vi "SetModelAndSuffix.vi"(5 "Revision":string, 6 "Serial Number":string, 7 "PartNumberData":T1(array[cluster]), 8 "error in (no error)":errorcluster, 9 "Part Number":string, 10 "ArrayIndex":i32=1, 11 "Sequence Context In":refnum<k7>) -> (0 "error out":errorcluster, 3 "Sequence Context Out":refnum<k7>)   [LabVIEW 2021]
uses:
  <vilib>/addons/TestStand/_TSUtility.llb/TestStand - Set Property Value (String).vi
  <vilib>/addons/TestStand/_TSUtility.llb/TestStand - Set Property Value (Boolean).vi
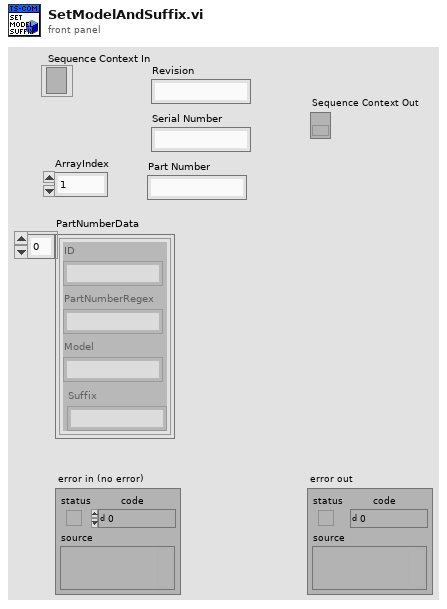
[diagram p1: front panel]
types:
  T1 = cluster{"ID":string, "PartNumberRegex":string, "Model":string, "Suffix":string}[]
  T2 = cluster{"ID":string, "PartNumberRegex":string, "Model":string, "Suffix":string}
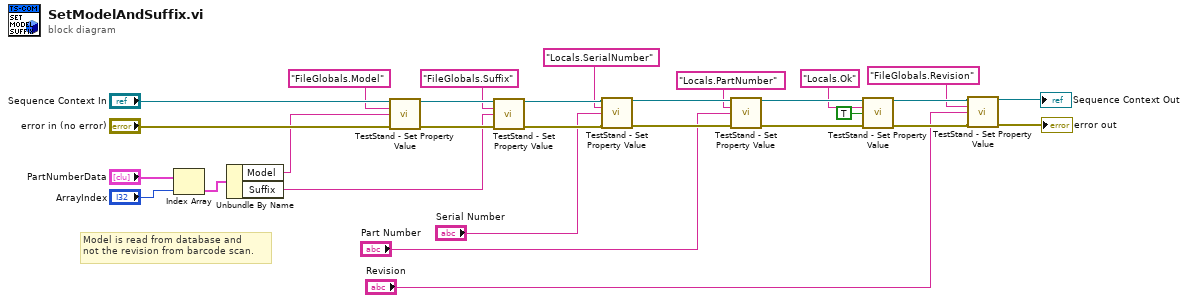
[diagram p0: block diagram]
diagram:
  # "Model is read from database and \nnot the revision from barcode scan."
  n1 = Index Array(array="PartNumberData", index="ArrayIndex") -> (element=w9:T2)
  n2 = Unbundle By Name(w9) -> ("Model"=w7:string, "Suffix"=w8:string)
  n3 = call-poly <vilib>:"TestStand - Set Property Value.vi"("Sequence Context In"="Sequence Context In", "Lookup String"="FileGlobals.Model", "New Value"=w7, "error in (no error)"="error in (no error)") -> ("Sequence Context Out"=w27:refnum<k7>, "error out"=w25:errorcluster)  [unwired: 10 in]
  n4 = call-poly <vilib>:"TestStand - Set Property Value.vi"("Sequence Context In"=w27, "Lookup String"="FileGlobals.Suffix", "New Value"=w8, "error in (no error)"=w25) -> ("Sequence Context Out"=w23:refnum<k7>, "error out"=w22:errorcluster)  [unwired: 10 in]
  n5 = call-poly <vilib>:"TestStand - Set Property Value.vi"("Sequence Context In"=w23, "Lookup String"="Locals.SerialNumber", "New Value"="Serial Number", "error in (no error)"=w22) -> ("Sequence Context Out"=w21:refnum<k7>, "error out"=w20:errorcluster)  [unwired: 10 in]
  n6 = call-poly <vilib>:"TestStand - Set Property Value.vi"("Sequence Context In"=w21, "Lookup String"="Locals.PartNumber", "New Value"="Part Number", "error in (no error)"=w20) -> ("Sequence Context Out"=w19:refnum<k7>, "error out"=w14:errorcluster)  [unwired: 10 in]
  n7 = call-poly <vilib>:"TestStand - Set Property Value.vi"("Sequence Context In"=w19, "Lookup String"="Locals.Ok", "New Value"=TRUE, "error in (no error)"=w14) -> ("Sequence Context Out"=w4:refnum<k7>, "error out"=w6:errorcluster)  [unwired: 10 in]
  n8 = call-poly <vilib>:"TestStand - Set Property Value.vi"("Sequence Context In"=w4, "Lookup String"="FileGlobals.Revision", "New Value"="Revision", "error in (no error)"=w6) -> ("Sequence Context Out"=→"Sequence Context Out":refnum<k7>, "error out"=→"error out":errorcluster)  [unwired: 10 in]
